vi "Run.vi"(8 "error in (no error)":errorcluster, 10 "반복":u32, 11 "Ch selection":T1) -> (0 "error out":errorcluster, 3 "stop":bool)   [LabVIEW 2019]
uses:
  _ctrl/rw.ctl
  cmd_runStop.ctl
  cmd_timer.ctl
  Durability/common/result.ctl
  _ctrl/init-r-stop.ctl
  Durability/common/Global 1.vi
  Glob_setting.vi
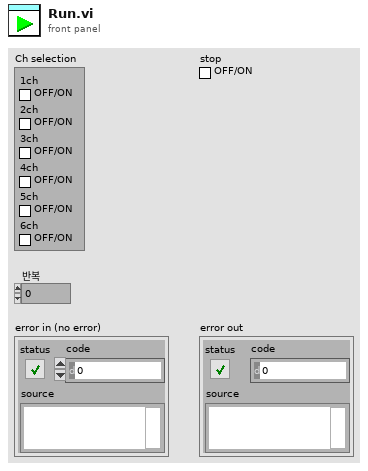
[diagram p1: front panel]
types:
  T1 = cluster{"1ch":bool, "2ch":bool, "3ch":bool, "4ch":bool, "5ch":bool, "6ch":bool}
  T2 = typedef "cmd_runStop.ctl" = enum16{"Init", "Run 1", "Stop", "Run 2", "Exit"}
  T3 = typedef "rw.ctl" = enum16{"read", "write"}
  T4 = typedef "cap_config.ctl" = cluster{"Test Mode":enum32{"6.3.2 저온 작동/방치 시험", "6.3.3 고온 작동/방치 시험", "6.3.4 온도 싸이클 시험", "6.3.6 온습도 싸이클 시험", "6.3.8 결로 시험", "6.3.9 빙결 시험"}, "ON time[ms]":dbl, "OFF time[ms]":dbl, "1. 작동시간[분]":dbl, "2. 미작동시간[분]":dbl, "3. 작동시간[분]":dbl, "level[V]":dbl, "duty":dbl, "Freq":dbl, "Voltage+[V]":dbl, "Voltage-[V]":dbl, "Current+[A]":dbl, "Current-[A]":dbl, "출력전압[V]":dbl, "출력전류[A]":dbl, "OVP Level":dbl, "OCP Level":dbl, "Time Div":u16, "Record Len":i32, "방전 기준[V]":dbl, "Repeate (Each Ch)":u32, "Cycle[N]":u32, "ON/OFF 회 수[N]":dbl, "TrigPos[%]":dbl, "시험시간[분]":dbl}
  T5 = enum32{"6.3.2 저온 작동/방치 시험", "6.3.3 고온 작동/방치 시험", "6.3.4 온도 싸이클 시험", "6.3.6 온습도 싸이클 시험", "6.3.8 결로 시험", "6.3.9 빙결 시험"}
  T6 = typedef "result.ctl" = enum16{"Init", "OK", "NG", "Shutdown", "Testing", "Completion", "Device Error", "Start", "작동", "미작동", "작동 대기", "작동 1"}
  T7 = typedef "cmd_timer.ctl" = enum16{"init", "init_update", "run", "default", "update"}
  T8 = typedef "init-r-stop.ctl" = enum16{"ini", "read", "stop"}
  T9 = typedef "rc-seq_enum.ctl" = enum16{"hw set", "Pwr-in on", "ch-relay on", "Pwr-out on", "AO on", "AO 0v", "Pwr-in off", "Relay-all off", "Pwr-out off", "Discharge", "950 read", "Run", "Stop"}
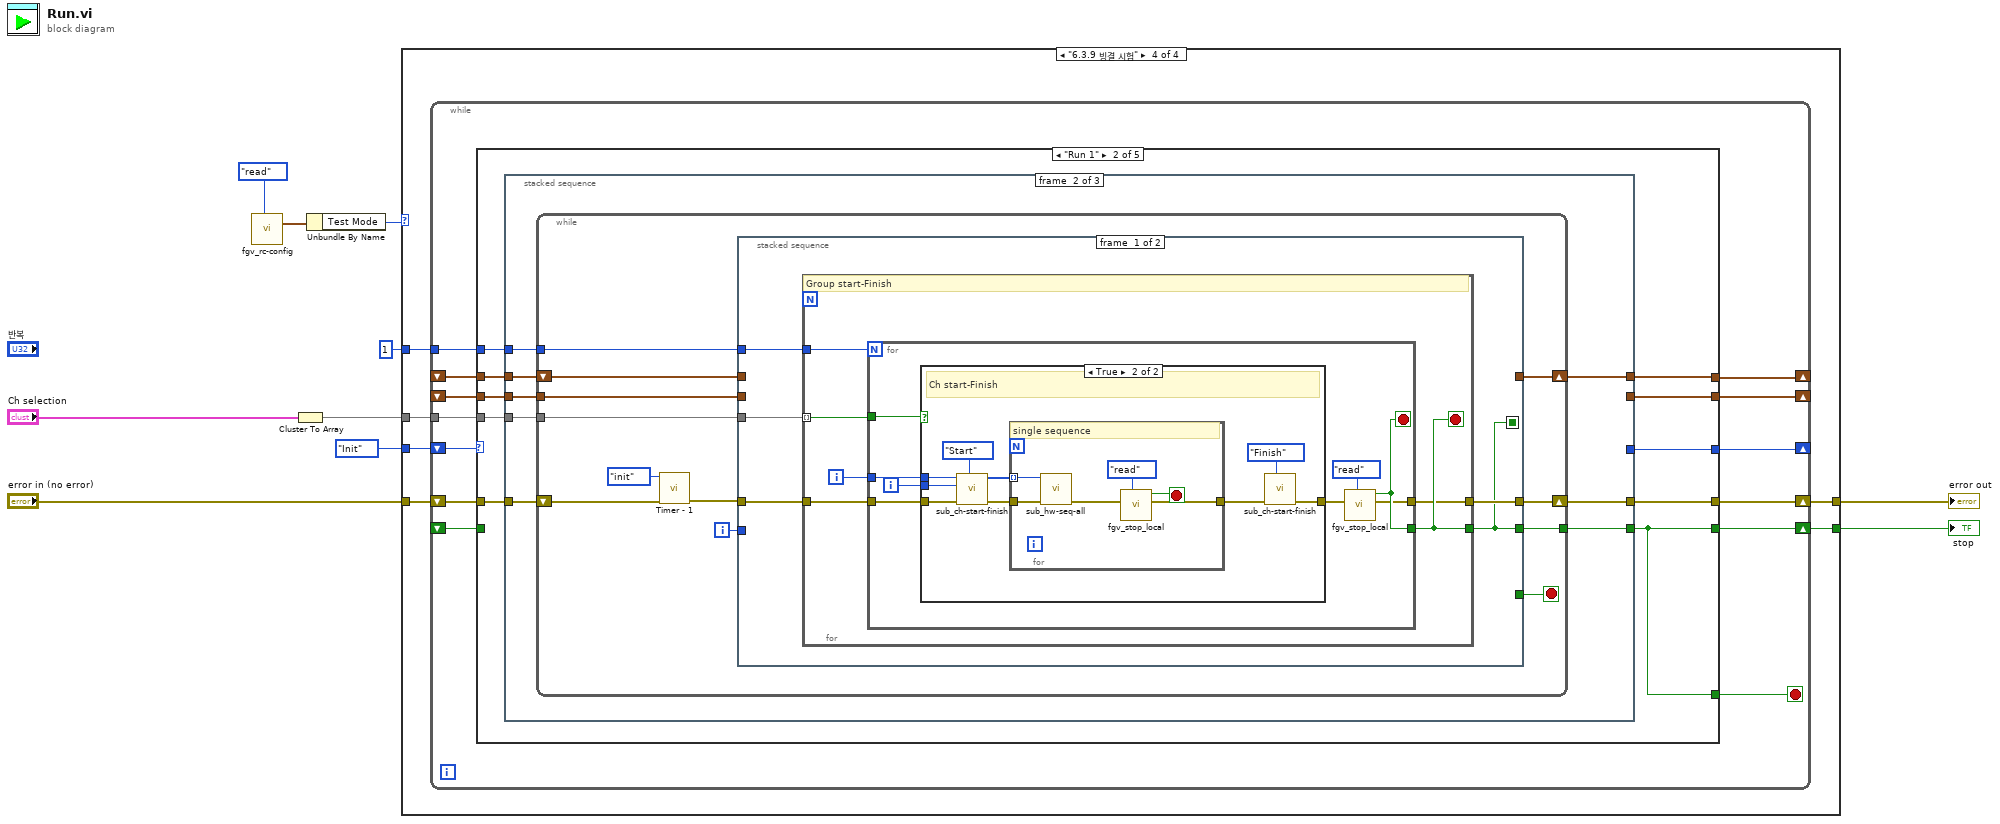
[diagram p0: block diagram]
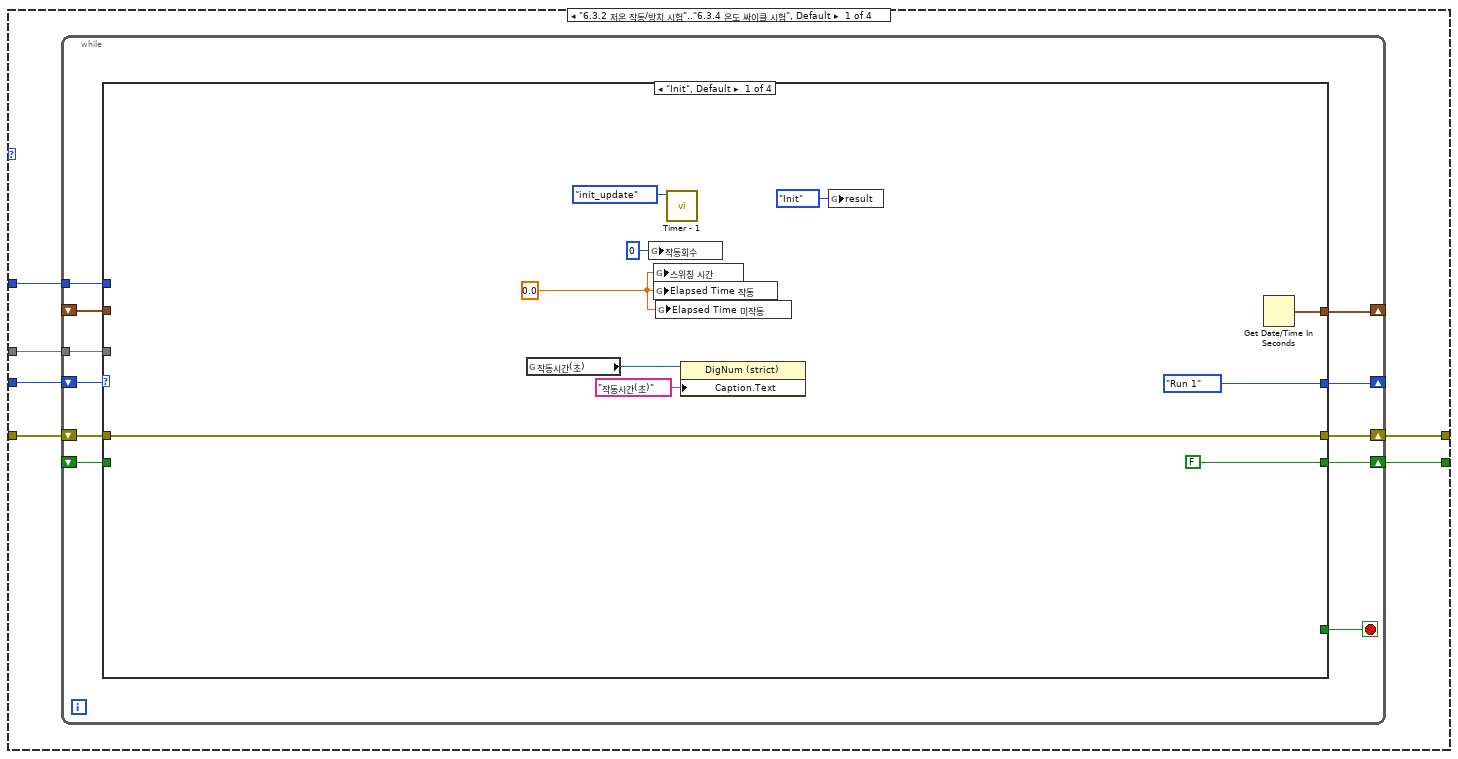
[diagram p2: hidden frame]
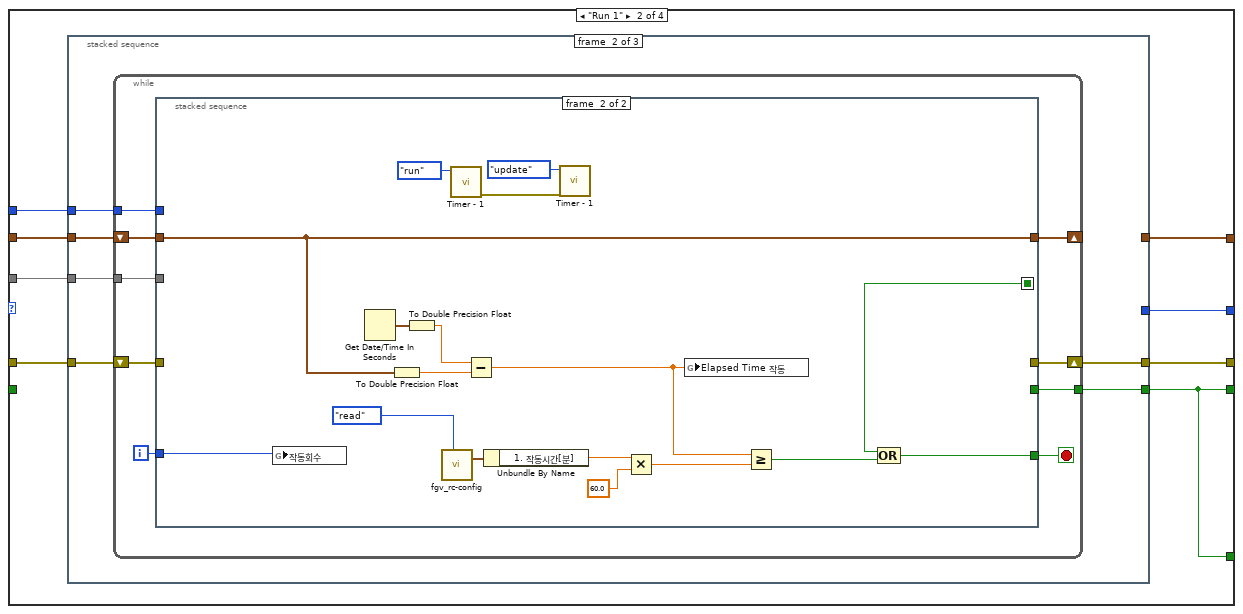
[diagram p3: hidden frame]
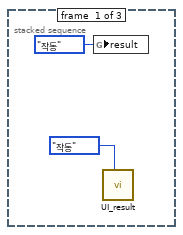
[diagram p4: hidden frame]
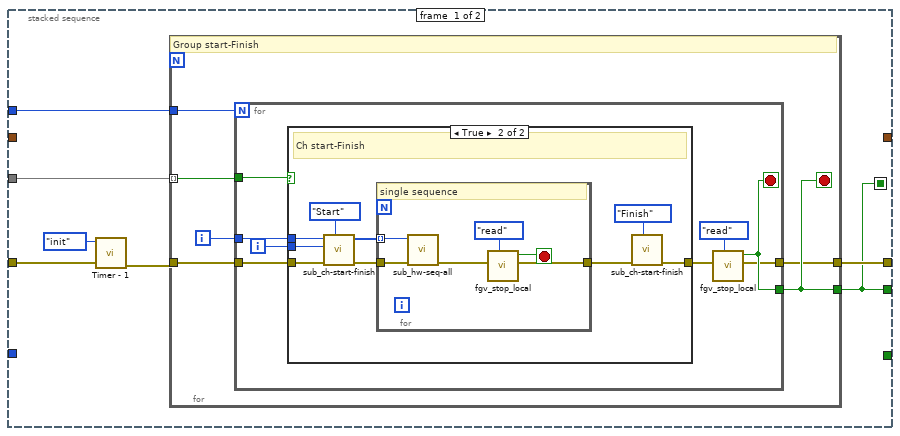
[diagram p5: hidden frame]
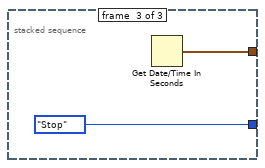
[diagram p7: hidden frame]
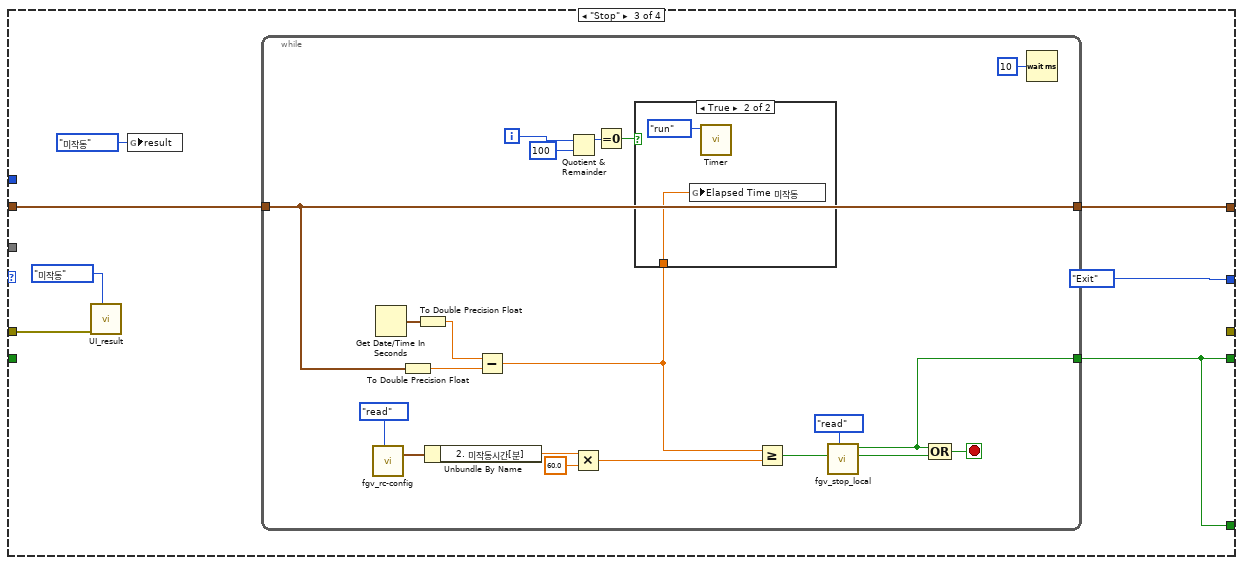
[diagram p8: hidden frame]
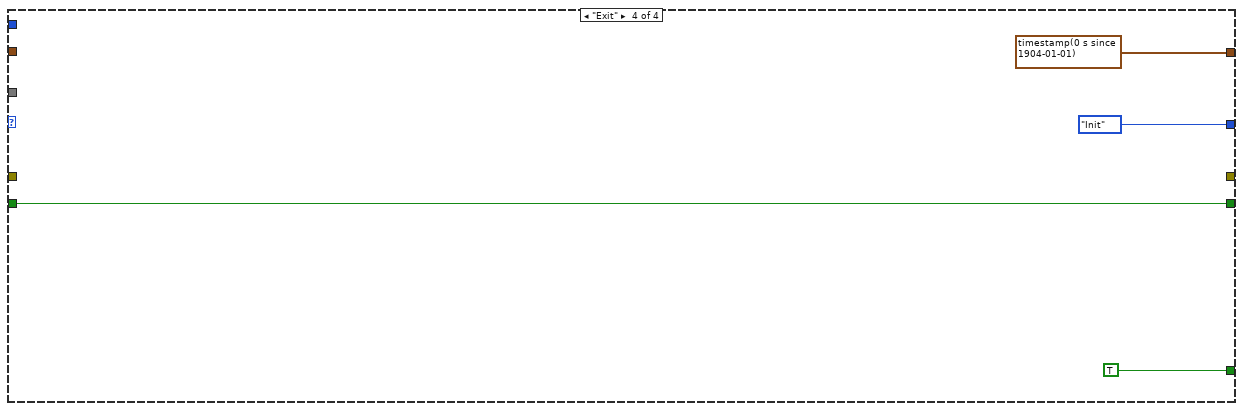
[diagram p10: hidden frame]
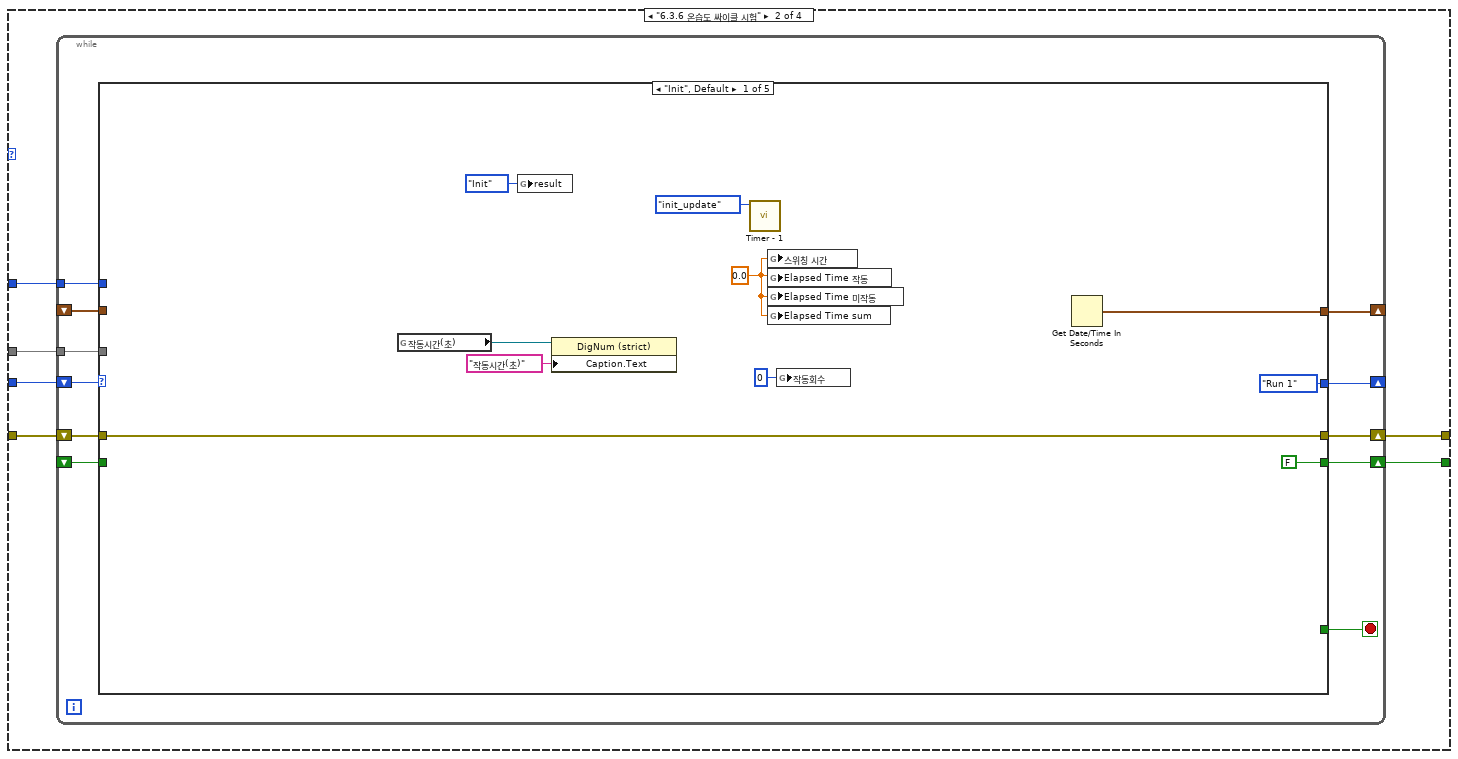
[diagram p11: hidden frame]
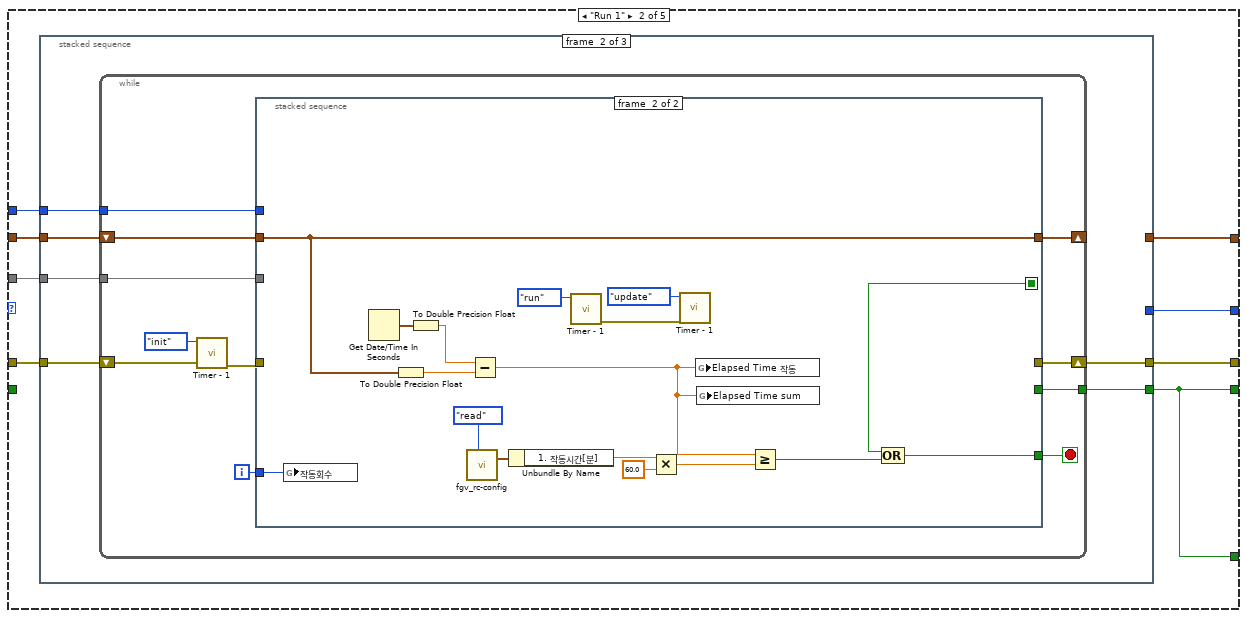
[diagram p12: hidden frame]
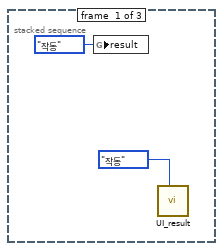
[diagram p13: hidden frame]
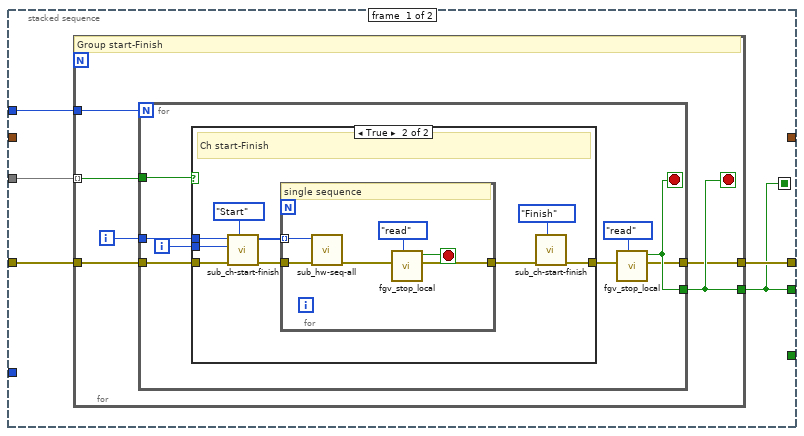
[diagram p14: hidden frame]
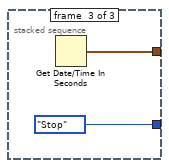
[diagram p16: hidden frame]
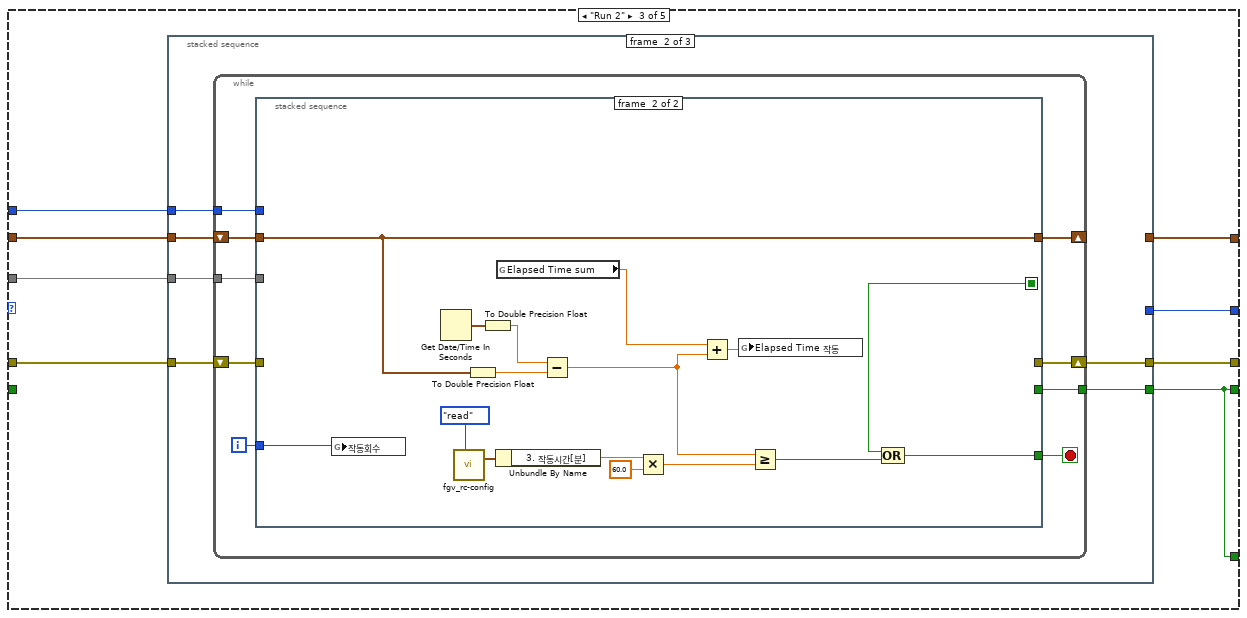
[diagram p17: hidden frame]
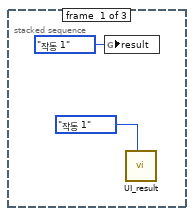
[diagram p18: hidden frame]
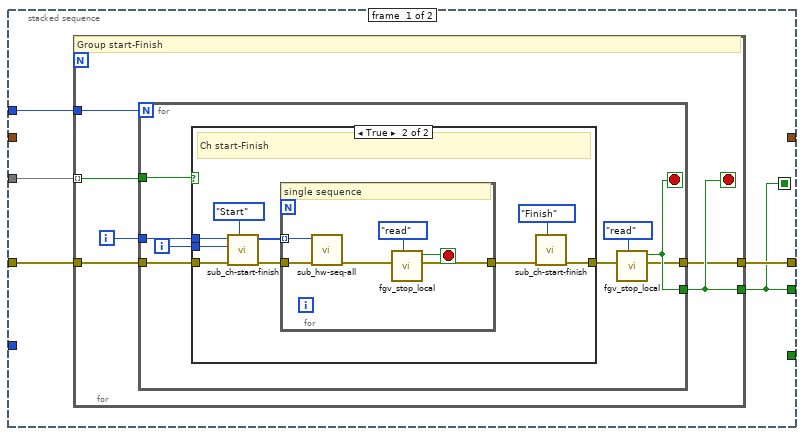
[diagram p19: hidden frame]
diagram:
  n1 = call "fgv_rc-config.vi"("cmd"=rw."read") -> ("Testconfig out"=w5:T4)  [unwired: 9 in, 1 out]
  n2 = Cluster To Array(cluster="Ch selection") -> (array=w6:bool[])
  n3 = Unbundle By Name(w5) -> ("Test Mode"=w3:T5)
  n4 = case shown="\"6.3.9 빙결 시험\"" w3 {
    tunnel: u32 1 ("반복") -> [w16 w156 w379 w637]
    tunnel: [w15 w155 w378 w636] -> w10
    tunnel: "error in (no error)" -> [w14 w154 w377 w635]
    tunnel: [w13 w153 w376 w634] -> w8
    tunnel: w6 -> [w12 w152 w375 w633]
    tunnel: cmd_runStop."Init" ("Enum") -> [w11 w151 w374 w632]
    frame "6.3.2 저온 작동/방치 시험".."6.3.4 온도 싸이클 시험", Default {
      n5 = while {
        tunnel: w16 -> [w27]
        tunnel: w12 -> [w23]
        shift-right: [w26] -> w15
        shift-left: w14 -> [w25]
        shift-right: [w21] -> _
        shift-left: _ -> [w20]
        shift-right: [w19] -> _
        shift-left: w11 -> [w22]
        shift-right: [w24] -> w13
        shift-left: _ -> [w18]
        stop <- w17 stop-if-true
        n6 = case shown="\"Init\", Default" w22 {
          tunnel: w27 -> [_ w45 _ _]
          tunnel: [w36 w44 _ _] -> w26
          tunnel: w25 -> [w36 w43 w121 _]
          tunnel: [FALSE ("stop") w38 w120 w148] -> w24
          tunnel: w23 -> [_ w42 _ _]
          tunnel: [w37 w40 w124 timestamp(0 s since 1904-01-01) ("seconds since 1Jan1904")] -> w21
          tunnel: w20 -> [_ w41 w125 _]
          tunnel: [cmd_runStop."Run 1" ("Enum") w39 cmd_runStop."Exit" ("Enum") cmd_runStop."Init" ("Enum")] -> w19
          tunnel: w18 -> [_ _ _ w148]
          tunnel: [_ w38 w120 TRUE] -> w17
          frame "Init", Default {
            w33 = 0.0 ("Elapsed Time")
            n7 = global read "Global 1.vi" "작동시간(초)"() -> (w31:refnum<vi>)
            n8 = global write "Global 1.vi" "작동회수"(0 ("작동회수")) -> ()
            n9 = global write "Global 1.vi" "스위칭 시간"(w33) -> ()
            n10 = global write "Global 1.vi" "Elapsed Time 작동"(w33) -> ()
            n11 = global write "Global 1.vi" "Elapsed Time 미작동"(w33) -> ()
            n12 = call "Timer - 1.vi"("cmd"=cmd_timer."init_update") -> ()  [unwired: 8 in, 3 out]
            n13 = property class="DigNum (strict)"(reference=w31, "Caption.Text"="작동시간(초)" ("Label.Text")) -> ()  [unwired: 1 in, 2 out]
            n14 = global write "Glob_setting.vi" "result"(result."Init" ("result")) -> ()
            n15 = Get Date/Time In Seconds() -> (seconds since 1Jan1904=w37:timestamp)
          }
          frame "Run 1" {
            n16 = stacked-sequence {
              tunnel: w45 -> [_ w53 _]
              tunnel: [_ w52 _] -> w44
              tunnel: w43 -> [_ w51 _]
              tunnel: [_ w50 _] -> w38
              tunnel: w42 -> [_ w49 _]
              tunnel: w41 -> [_ w48 _]
              tunnel: [_ _ w117] -> w40
              tunnel: [_ _ cmd_runStop."Stop" ("Enum")] -> w39
              frame #0 {
                n17 = global write "Glob_setting.vi" "result"(result."작동" ("result")) -> ()
                n18 = call "UI_result.vi"("result"=result."작동") -> ()  [unwired: 10 in, 1 out]
              }
              frame #1 {
                n19 = while {
                  tunnel: w53 -> [w62]
                  tunnel: [w59] -> w50
                  tunnel: w49 -> [w58]
                  shift-right: [w61] -> w52
                  shift-left: w51 -> [w60]
                  shift-right: [w55] -> _
                  shift-left: w48 -> [w57]
                  i -> [w54]
                  stop <- w56 stop-if-true
                  n20 = stacked-sequence {
                    seq-local: [w66 _] -> [_ w111]
                    tunnel: w62 -> [w69 _]
                    tunnel: [w68 _] -> w61
                    tunnel: w60 -> [w64 _]
                    tunnel: [w66 _] -> w59
                    tunnel: w58 -> [w67 _]
                    tunnel: w57 -> [_ w108]
                    tunnel: [_ w109] -> w56
                    tunnel: [_ w108] -> w55
                    tunnel: w54 -> [_ w104]
                    frame #0 {
                      n21 = call "Timer - 1.vi"("error in (no error)"=w64, "cmd"=cmd_timer."init") -> ("error out"=w63:errorcluster)  [unwired: 7 in, 2 out]
                      n22 = for {
                        tunnel: [w73] -> w66
                        tunnel: w67 -> [w75] mode=indexing
                        tunnel: w63 -> [w71]
                        tunnel: [w72] -> w68
                        tunnel: w69 -> [w70]
                        i -> [w74]
                        stop <- w73 stop-if-true
                        # "Group start-Finish"
                        n23 = for {
                          N: w70 -> [_]
                          tunnel: w74 -> [w82]
                          tunnel: w71 -> [w81]
                          tunnel: [w76] -> w72
                          tunnel: w75 -> [w83]
                          tunnel: [w77] -> w73
                          i -> [w80]
                          stop <- w77 stop-if-true
                          n24 = case shown="True" w83 {
                            tunnel: w82 -> [_ w92]
                            tunnel: [w84 w85] -> w78
                            tunnel: w81 -> [w84 w87]
                            tunnel: w80 -> [_ w86]
                            frame False {
                            }
                            frame True {
                              # "Ch start-Finish"
                              n25 = call "sub_ch-start-finish.vi"("cmd"=enum16{"Start", "Finish"}."Start", "error in"=w87, "repeat"=w86, "Ch"=w92) -> ("error out"=w93:errorcluster, "HWseq-array"=w90:T9[])  [unwired: 5 in, 1 out]
                              n26 = for {
                                tunnel: w90 -> [w97] mode=indexing
                                tunnel: w93 -> [w94]
                                tunnel: [w95] -> w88
                                stop <- w98 stop-if-true
                                # "single sequence"
                                n27 = call "sub_hw-seq-all.vi"("error"=w94, "HWseq"=w97) -> ("error out"=w96:errorcluster)  [unwired: 9 in]
                                n28 = call "fgv_stop_local.vi"("cmd"=init-r-stop."read", "error in (no error)"=w96) -> ("error out"=w95:errorcluster, "stop"=w98:bool)  [unwired: 8 in]
                              }
                              n29 = call "sub_ch-start-finish.vi"("cmd"=enum16{"Start", "Finish"}."Finish", "error in"=w88) -> ("error out"=w85:errorcluster)  [unwired: 7 in, 2 out]
                            }
                          }
                          n30 = call "fgv_stop_local.vi"("cmd"=init-r-stop."read", "error in (no error)"=w78) -> ("error out"=w76:errorcluster, "stop"=w77:bool)  [unwired: 8 in]
                        }
                      }
                    }
                    frame #1 {
                      n31 = global write "Global 1.vi" "작동회수"(w104) -> ()
                      n32 = Get Date/Time In Seconds() -> (seconds since 1Jan1904=w116:timestamp)
                      n33 = To Double Precision Float(number=w108) -> (double precision float=w114:dbl)
                      n34 = To Double Precision Float(number=w116) -> (double precision float=w115:dbl)
                      n35 = call "fgv_rc-config.vi"("cmd"=rw."read") -> ("Testconfig out"=w113:T4)  [unwired: 9 in, 1 out]
                      n36 = call "Timer - 1.vi"("cmd"=cmd_timer."run") -> ("error out"=w100:errorcluster)  [unwired: 8 in, 2 out]
                      n37 = Subtract(x=w115, y=w114) -> (x-y=w103:dbl)
                      n38 = Unbundle By Name(w113) -> ("1. 작동시간[분]"=w107:dbl)
                      n39 = call "Timer - 1.vi"("error in (no error)"=w100, "cmd"=cmd_timer."update") -> ()  [unwired: 7 in, 3 out]
                      n40 = Multiply(x=w107, y=60.0) -> (x*y=w105:dbl)
                      n41 = global write "Global 1.vi" "Elapsed Time 작동"(w103) -> ()
                      n42 = Greater Or Equal?(x=w103, y=w105) -> (x >= y?=w110:bool)
                      n43 = Compound Arithmetic op=OR(w111, w110) -> (w109:bool)
                    }
                  }
                }
              }
              frame #2 {
                n44 = Get Date/Time In Seconds() -> (seconds since 1Jan1904=w117:timestamp)
              }
            }
          }
          frame "Stop" {
            n45 = call "UI_result.vi"("result"=result."미작동", "error in (no error)"=w121) -> ()  [unwired: 9 in, 1 out]
            n46 = global write "Glob_setting.vi" "result"(result."미작동" ("result")) -> ()
            n47 = while {
              tunnel: w125 -> [w132]
              tunnel: [w132] -> w124
              tunnel: [w131] -> w120
              i -> [w127]
              stop <- w133 stop-if-true
              n48 = call "fgv_rc-config.vi"("cmd"=rw."read") -> ("Testconfig out"=w139:T4)  [unwired: 9 in, 1 out]
              n49 = Get Date/Time In Seconds() -> (seconds since 1Jan1904=w142:timestamp)
              n50 = To Double Precision Float(number=w132) -> (double precision float=w140:dbl)
              n51 = To Double Precision Float(number=w142) -> (double precision float=w141:dbl)
              n52 = Unbundle By Name(w139) -> ("2. 미작동시간[분]"=w137:dbl)
              n53 = Subtract(x=w141, y=w140) -> (x-y=w126:dbl)
              n54 = Quotient & Remainder(x=w127, y=100) -> (x-y*floor(x/y)=w129:i32)  [unwired: 1 out]
              n55 = Multiply(x=w137, y=60.0) -> (x*y=w135:dbl)
              n56 = Equal To 0?(x=w129) -> (x = 0?=w128:bool)
              n57 = case shown="True" w128 {
                tunnel: w126 -> [_ w145]
                frame False {
                }
                frame True {
                  n58 = global write "Global 1.vi" "Elapsed Time 미작동"(w145) -> ()
                  n59 = call "Timer.vi"("cmd"=cmd_timer."run") -> ()  [unwired: 8 in, 3 out]
                }
              }
              n60 = Greater Or Equal?(x=w126, y=w135) -> (x >= y?=w134:bool)
              n61 = call "fgv_stop_local.vi"("cmd"=init-r-stop."read") -> ("stop"=w131:bool)  [unwired: 9 in, 1 out]
              n62 = Compound Arithmetic op=OR(w131, w134) -> (w133:bool)
              n63 = Wait (ms)(milliseconds to wait=u32 10) -> ()  [unwired: 1 out]
            }
          }
          frame "Exit" {
          }
        }
      }
    }
    frame "6.3.6 온습도 싸이클 시험" {
      n64 = while {
        tunnel: w156 -> [w167]
        tunnel: w152 -> [w163]
        shift-right: [w166] -> w155
        shift-left: w154 -> [w165]
        shift-right: [w161] -> _
        shift-left: _ -> [w160]
        shift-right: [w159] -> _
        shift-left: w151 -> [w162]
        shift-right: [w164] -> w153
        shift-left: _ -> [w158]
        stop <- w157 stop-if-true
        n65 = case shown="\"Init\", Default" w162 {
          tunnel: w167 -> [_ w185 w266 _ _]
          tunnel: [w176 w184 w265 _ _] -> w166
          tunnel: w165 -> [w176 w183 w264 w339 _]
          tunnel: [FALSE ("stop") w178 w259 w338 w371] -> w164
          tunnel: w163 -> [_ w182 w263 _ _]
          tunnel: [w177 w180 w261 w342 timestamp(0 s since 1904-01-01) ("seconds since 1Jan1904")] -> w161
          tunnel: w160 -> [_ w181 w262 w343 _]
          tunnel: [cmd_runStop."Run 1" ("Enum") w179 w260 w341 cmd_runStop."Init" ("Enum")] -> w159
          tunnel: w158 -> [_ _ _ _ w371]
          tunnel: [_ w178 w259 w338 TRUE] -> w157
          frame "Init", Default {
            w168 = 0.0 ("Elapsed Time")
            n66 = global read "Global 1.vi" "작동시간(초)"() -> (w172:refnum<vi>)
            n67 = global write "Glob_setting.vi" "result"(result."Init" ("result")) -> ()
            n68 = property class="DigNum (strict)"(reference=w172, "Caption.Text"="작동시간(초)" ("Label.Text")) -> ()  [unwired: 1 in, 2 out]
            n69 = call "Timer - 1.vi"("cmd"=cmd_timer."init_update") -> ()  [unwired: 8 in, 3 out]
            n70 = global write "Global 1.vi" "스위칭 시간"(w168) -> ()
            n71 = global write "Global 1.vi" "Elapsed Time 작동"(w168) -> ()
            n72 = global write "Global 1.vi" "Elapsed Time 미작동"(w168) -> ()
            n73 = global write "Global 1.vi" "Elapsed Time sum"(w168) -> ()
            n74 = global write "Global 1.vi" "작동회수"(0 ("작동회수")) -> ()
            n75 = Get Date/Time In Seconds() -> (seconds since 1Jan1904=w177:timestamp)
          }
          frame "Run 1" {
            n76 = stacked-sequence {
              tunnel: w185 -> [_ w193 _]
              tunnel: [_ w192 _] -> w184
              tunnel: w183 -> [_ w191 _]
              tunnel: [_ w190 _] -> w178
              tunnel: w182 -> [_ w189 _]
              tunnel: w181 -> [_ w188 _]
              tunnel: [_ _ w257] -> w180
              tunnel: [_ _ cmd_runStop."Stop" ("Enum")] -> w179
              frame #0 {
                n77 = global write "Glob_setting.vi" "result"(result."작동" ("result")) -> ()
                n78 = call "UI_result.vi"("result"=result."작동") -> ()  [unwired: 10 in, 1 out]
              }
              frame #1 {
                n79 = while {
                  tunnel: w193 -> [w204]
                  tunnel: [w202] -> w190
                  tunnel: w189 -> [w201]
                  shift-right: [w203] -> w192
                  shift-left: w191 -> [w195]
                  shift-right: [w198] -> _
                  shift-left: w188 -> [w200]
                  i -> [w197]
                  stop <- w199 stop-if-true
                  n80 = call "Timer - 1.vi"("error in (no error)"=w195, "cmd"=cmd_timer."init") -> ("error out"=w194:errorcluster)  [unwired: 7 in, 2 out]
                  n81 = stacked-sequence {
                    seq-local: [w205 _] -> [_ w251]
                    tunnel: w204 -> [w209 _]
                    tunnel: [w208 _] -> w203
                    tunnel: w194 -> [w207 _]
                    tunnel: [w205 _] -> w202
                    tunnel: w201 -> [w206 _]
                    tunnel: w200 -> [_ w248]
                    tunnel: [_ w249] -> w199
                    tunnel: [_ w248] -> w198
                    tunnel: w197 -> [_ w244]
                    frame #0 {
                      n82 = for {
                        tunnel: [w213] -> w205
                        tunnel: w206 -> [w215] mode=indexing
                        tunnel: w207 -> [w211]
                        tunnel: [w212] -> w208
                        tunnel: w209 -> [w210]
                        i -> [w214]
                        stop <- w213 stop-if-true
                        # "Group start-Finish"
                        n83 = for {
                          N: w210 -> [_]
                          tunnel: w214 -> [w222]
                          tunnel: w211 -> [w221]
                          tunnel: [w216] -> w212
                          tunnel: w215 -> [w223]
                          tunnel: [w217] -> w213
                          i -> [w220]
                          stop <- w217 stop-if-true
                          n84 = case shown="True" w223 {
                            tunnel: w222 -> [_ w232]
                            tunnel: [w224 w225] -> w218
                            tunnel: w221 -> [w224 w227]
                            tunnel: w220 -> [_ w226]
                            frame False {
                            }
                            frame True {
                              # "Ch start-Finish"
                              n85 = call "sub_ch-start-finish.vi"("cmd"=enum16{"Start", "Finish"}."Start", "error in"=w227, "repeat"=w226, "Ch"=w232) -> ("error out"=w233:errorcluster, "HWseq-array"=w230:T9[])  [unwired: 5 in, 1 out]
                              n86 = for {
                                tunnel: w230 -> [w237] mode=indexing
                                tunnel: w233 -> [w234]
                                tunnel: [w235] -> w228
                                stop <- w238 stop-if-true
                                # "single sequence"
                                n87 = call "sub_hw-seq-all.vi"("error"=w234, "HWseq"=w237) -> ("error out"=w236:errorcluster)  [unwired: 9 in]
                                n88 = call "fgv_stop_local.vi"("cmd"=init-r-stop."read", "error in (no error)"=w236) -> ("error out"=w235:errorcluster, "stop"=w238:bool)  [unwired: 8 in]
                              }
                              n89 = call "sub_ch-start-finish.vi"("cmd"=enum16{"Start", "Finish"}."Finish", "error in"=w228) -> ("error out"=w225:errorcluster)  [unwired: 7 in, 2 out]
                            }
                          }
                          n90 = call "fgv_stop_local.vi"("cmd"=init-r-stop."read", "error in (no error)"=w218) -> ("error out"=w216:errorcluster, "stop"=w217:bool)  [unwired: 8 in]
                        }
                      }
                    }
                    frame #1 {
                      n91 = global write "Global 1.vi" "작동회수"(w244) -> ()
                      n92 = Get Date/Time In Seconds() -> (seconds since 1Jan1904=w256:timestamp)
                      n93 = To Double Precision Float(number=w248) -> (double precision float=w254:dbl)
                      n94 = To Double Precision Float(number=w256) -> (double precision float=w255:dbl)
                      n95 = call "fgv_rc-config.vi"("cmd"=rw."read") -> ("Testconfig out"=w253:T4)  [unwired: 9 in, 1 out]
                      n96 = Subtract(x=w255, y=w254) -> (x-y=w240:dbl)
                      n97 = Unbundle By Name(w253) -> ("1. 작동시간[분]"=w247:dbl)
                      n98 = call "Timer - 1.vi"("cmd"=cmd_timer."run") -> ("error out"=w241:errorcluster)  [unwired: 8 in, 2 out]
                      n99 = Multiply(x=w247, y=60.0) -> (x*y=w245:dbl)
                      n100 = call "Timer - 1.vi"("error in (no error)"=w241, "cmd"=cmd_timer."update") -> ()  [unwired: 7 in, 3 out]
                      n101 = global write "Global 1.vi" "Elapsed Time 작동"(w240) -> ()
                      n102 = global write "Global 1.vi" "Elapsed Time sum"(w240) -> ()
                      n103 = Greater Or Equal?(x=w240, y=w245) -> (x >= y?=w250:bool)
                      n104 = Compound Arithmetic op=OR(w251, w250) -> (w249:bool)
                    }
                  }
                }
              }
              frame #2 {
                n105 = Get Date/Time In Seconds() -> (seconds since 1Jan1904=w257:timestamp)
              }
            }
          }
          frame "Run 2" {
            n106 = stacked-sequence {
              tunnel: w266 -> [_ w274 _]
              tunnel: [_ w273 _] -> w265
              tunnel: w264 -> [_ w272 _]
              tunnel: [_ w271 _] -> w259
              tunnel: w263 -> [_ w270 _]
              tunnel: w262 -> [_ w269 _]
              tunnel: [_ _ w335] -> w261
              tunnel: [_ _ cmd_runStop."Exit" ("Enum")] -> w260
              frame #0 {
                n107 = global write "Glob_setting.vi" "result"(result."작동 1" ("result")) -> ()
                n108 = call "UI_result.vi"("result"=result."작동 1") -> ()  [unwired: 10 in, 1 out]
              }
              frame #1 {
                n109 = while {
                  tunnel: w274 -> [w283]
                  tunnel: [w280] -> w271
                  tunnel: w270 -> [w279]
                  shift-right: [w282] -> w273
                  shift-left: w272 -> [w281]
                  shift-right: [w276] -> _
                  shift-left: w269 -> [w278]
                  i -> [w275]
                  stop <- w277 stop-if-true
                  n110 = stacked-sequence {
                    seq-local: [w284 _] -> [_ w329]
                    tunnel: w283 -> [w288 _]
                    tunnel: [w287 _] -> w282
                    tunnel: w281 -> [w286 _]
                    tunnel: [w284 _] -> w280
                    tunnel: w279 -> [w285 _]
                    tunnel: w278 -> [_ w326]
                    tunnel: [_ w327] -> w277
                    tunnel: [_ w326] -> w276
                    tunnel: w275 -> [_ w322]
                    frame #0 {
                      n111 = for {
                        tunnel: [w292] -> w284
                        tunnel: w285 -> [w294] mode=indexing
                        tunnel: w286 -> [w290]
                        tunnel: [w291] -> w287
                        tunnel: w288 -> [w289]
                        i -> [w293]
                        stop <- w292 stop-if-true
                        # "Group start-Finish"
                        n112 = for {
                          N: w289 -> [_]
                          tunnel: w293 -> [w301]
                          tunnel: w290 -> [w300]
                          tunnel: [w295] -> w291
                          tunnel: w294 -> [w302]
                          tunnel: [w296] -> w292
                          i -> [w299]
                          stop <- w296 stop-if-true
                          n113 = case shown="True" w302 {
                            tunnel: w301 -> [_ w311]
                            tunnel: [w303 w304] -> w297
                            tunnel: w300 -> [w303 w306]
                            tunnel: w299 -> [_ w305]
                            frame False {
                            }
                            frame True {
                              # "Ch start-Finish"
                              n114 = call "sub_ch-start-finish.vi"("cmd"=enum16{"Start", "Finish"}."Start", "error in"=w306, "repeat"=w305, "Ch"=w311) -> ("error out"=w312:errorcluster, "HWseq-array"=w309:T9[])  [unwired: 5 in, 1 out]
                              n115 = for {
                                tunnel: w309 -> [w316] mode=indexing
                                tunnel: w312 -> [w313]
                                tunnel: [w314] -> w307
                                stop <- w317 stop-if-true
                                # "single sequence"
                                n116 = call "sub_hw-seq-all.vi"("error"=w313, "HWseq"=w316) -> ("error out"=w315:errorcluster)  [unwired: 9 in]
                                n117 = call "fgv_stop_local.vi"("cmd"=init-r-stop."read", "error in (no error)"=w315) -> ("error out"=w314:errorcluster, "stop"=w317:bool)  [unwired: 8 in]
                              }
                              n118 = call "sub_ch-start-finish.vi"("cmd"=enum16{"Start", "Finish"}."Finish", "error in"=w307) -> ("error out"=w304:errorcluster)  [unwired: 7 in, 2 out]
                            }
                          }
                          n119 = call "fgv_stop_local.vi"("cmd"=init-r-stop."read", "error in (no error)"=w297) -> ("error out"=w295:errorcluster, "stop"=w296:bool)  [unwired: 8 in]
                        }
                      }
                    }
                    frame #1 {
                      n120 = global write "Global 1.vi" "작동회수"(w322) -> ()
                      n121 = Get Date/Time In Seconds() -> (seconds since 1Jan1904=w334:timestamp)
                      n122 = call "fgv_rc-config.vi"("cmd"=rw."read") -> ("Testconfig out"=w331:T4)  [unwired: 9 in, 1 out]
                      n123 = To Double Precision Float(number=w326) -> (double precision float=w332:dbl)
                      n124 = To Double Precision Float(number=w334) -> (double precision float=w333:dbl)
                      n125 = Unbundle By Name(w331) -> ("3. 작동시간[분]"=w325:dbl)
                      n126 = global read "Global 1.vi" "Elapsed Time sum"() -> (w320:dbl)
                      n127 = Subtract(x=w333, y=w332) -> (x-y=w321:dbl)
                      n128 = Multiply(x=w325, y=60.0) -> (x*y=w323:dbl)
                      n129 = Add(x=w320, y=w321) -> (x+y=w319:dbl)
                      n130 = global write "Global 1.vi" "Elapsed Time 작동"(w319) -> ()
                      n131 = Greater Or Equal?(x=w321, y=w323) -> (x >= y?=w328:bool)
                      n132 = Compound Arithmetic op=OR(w329, w328) -> (w327:bool)
                    }
                  }
                }
              }
              frame #2 {
                n133 = Get Date/Time In Seconds() -> (seconds since 1Jan1904=w335:timestamp)
              }
            }
          }
          frame "Stop" {
            n134 = global write "Glob_setting.vi" "result"(result."미작동" ("result")) -> ()
            n135 = call "UI_result.vi"("result"=result."미작동", "error in (no error)"=w339) -> ()  [unwired: 9 in, 1 out]
            n136 = stacked-sequence {
              tunnel: w343 -> [w345 _]
              tunnel: [_ w368] -> w342
              tunnel: [w344 _] -> w338
              tunnel: [_ cmd_runStop."Run 2" ("Enum")] -> w341
              frame #0 {
                n137 = while {
                  tunnel: [w351] -> w344
                  shift-right: [w352] -> _
                  shift-left: w345 -> [w352]
                  i -> [w347]
                  stop <- w353 stop-if-true
                  n138 = call "fgv_rc-config.vi"("cmd"=rw."read") -> ("Testconfig out"=w359:T4)  [unwired: 9 in, 1 out]
                  n139 = Get Date/Time In Seconds() -> (seconds since 1Jan1904=w362:timestamp)
                  n140 = To Double Precision Float(number=w352) -> (double precision float=w360:dbl)
                  n141 = To Double Precision Float(number=w362) -> (double precision float=w361:dbl)
                  n142 = Unbundle By Name(w359) -> ("2. 미작동시간[분]"=w357:dbl)
                  n143 = Quotient & Remainder(x=w347, y=100) -> (x-y*floor(x/y)=w349:i32)  [unwired: 1 out]
                  n144 = Subtract(x=w361, y=w360) -> (x-y=w346:dbl)
                  n145 = Equal To 0?(x=w349) -> (x = 0?=w348:bool)
                  n146 = case shown="True" w348 {
                    tunnel: w346 -> [_ w365]
                    frame False {
                    }
                    frame True {
                      n147 = global write "Global 1.vi" "Elapsed Time 미작동"(w365) -> ()
                      n148 = call "Timer.vi"("cmd"=cmd_timer."run") -> ()  [unwired: 8 in, 3 out]
                    }
                  }
                  n149 = Multiply(x=w357, y=60.0) -> (x*y=w355:dbl)
                  n150 = Greater Or Equal?(x=w346, y=w355) -> (x >= y?=w354:bool)
                  n151 = call "fgv_stop_local.vi"("cmd"=init-r-stop."read") -> ("stop"=w351:bool)  [unwired: 9 in, 1 out]
                  n152 = Compound Arithmetic op=OR(w351, w354) -> (w353:bool)
                  n153 = Wait (ms)(milliseconds to wait=u32 10) -> ()  [unwired: 1 out]
                }
              }
              frame #1 {
                n154 = disable-structure shown="Disabled" {
                  frame Disabled {
                    n155 = global write "Global 1.vi" "Elapsed Time 작동"(0.0 ("Elapsed Time")) -> ()
                  }
                  frame Enabled {
                  }
                }
                n156 = Get Date/Time In Seconds() -> (seconds since 1Jan1904=w368:timestamp)
              }
            }
          }
          frame "Exit" {
          }
        }
      }
    }
    frame "6.3.8 결로 시험" {
      n157 = while {
        tunnel: w379 -> [w392]
        tunnel: w375 -> [w388]
        shift-right: [w391] -> w378
        shift-left: w377 -> [w390]
        shift-right: [w386] -> _
        shift-left: _ -> [w385]
        shift-right: [w384] -> _
        shift-left: w374 -> [w387]
        shift-right: [w389] -> w376
        shift-left: _ -> [w383]
        shift-right: [w381] -> _
        shift-left: _ -> [w380]
        stop <- w382 stop-if-true
        n158 = case shown="\"Stop\"" w387 {
          tunnel: w392 -> [_ w414 w501 _ _]
          tunnel: [w402 w413 w500 _ _] -> w391
          tunnel: w390 -> [w402 w404 w499 w577 _]
          tunnel: [FALSE ("stop") w406 w492 w576 w630] -> w389
          tunnel: w388 -> [_ w412 w498 _ _]
          tunnel: [w399 w410 w496 w582 w628] -> w386
          tunnel: w385 -> [_ w411 w497 w583 _]
          tunnel: [cmd_runStop."Run 1" ("Enum") w409 w495 w581 cmd_runStop."Init" ("Enum")] -> w384
          tunnel: w383 -> [_ _ _ _ w630]
          tunnel: [_ w406 w492 w576 TRUE] -> w382
          tunnel: [w399 w407 w494 w579 w628] -> w381
          tunnel: w380 -> [_ w408 w493 w580 _]
          frame "Init", Default {
            w393 = 0.0 ("Elapsed Time")
            n159 = global write "Glob_setting.vi" "result"(result."Init" ("result")) -> ()
            n160 = global read "Global 1.vi" "작동시간(초)"() -> (w397:refnum<vi>)
            n161 = global write "Global 1.vi" "작동회수"(0 ("작동회수")) -> ()
            n162 = global write "Global 1.vi" "스위칭 시간"(w393) -> ()
            n163 = global write "Global 1.vi" "Elapsed Time 작동"(w393) -> ()
            n164 = global write "Global 1.vi" "Elapsed Time 미작동"(w393) -> ()
            n165 = global write "Global 1.vi" "ETime 작동대기"(w393) -> ()
            n166 = property class="DigNum (strict)"(reference=w397, "Caption.Text"="작동경과 시간(초)" ("Label.Text")) -> ()  [unwired: 1 in, 2 out]
            n167 = call "Timer - 1.vi"("cmd"=cmd_timer."init_update") -> ()  [unwired: 8 in, 3 out]
            n168 = Get Date/Time In Seconds() -> (seconds since 1Jan1904=w399:timestamp)
          }
          frame "Run 1" {
            n169 = call "Timer - 1.vi"("error in (no error)"=w404, "cmd"=cmd_timer."init") -> ("error out"=w403:errorcluster)  [unwired: 7 in, 2 out]
            n170 = stacked-sequence {
              tunnel: w414 -> [_ w424 _]
              tunnel: [_ w423 _] -> w413
              tunnel: w403 -> [_ w422 _]
              tunnel: [_ w421 _] -> w406
              tunnel: w412 -> [_ w420 _]
              tunnel: w411 -> [_ w419 _]
              tunnel: [_ w418 _] -> w410
              tunnel: [_ _ cmd_runStop."Stop" ("Enum")] -> w409
              tunnel: w408 -> [_ w417 w490]
              tunnel: [_ _ w490] -> w407
              frame #0 {
                n171 = global write "Glob_setting.vi" "result"(result."작동" ("result")) -> ()
                n172 = call "UI_result.vi"("result"=result."작동") -> ()  [unwired: 10 in, 1 out]
              }
              frame #1 {
                n173 = while {
                  tunnel: w424 -> [w434]
                  tunnel: [w431] -> w421
                  tunnel: w420 -> [w430]
                  shift-right: [w433] -> w423
                  shift-left: w422 -> [w432]
                  shift-right: [w427] -> w418
                  shift-left: w419 -> [w429]
                  tunnel: w417 -> [w425]
                  i -> [w426]
                  stop <- w428 stop-if-true
                  n174 = stacked-sequence {
                    seq-local: [w435 _] -> [_ w481]
                    tunnel: w434 -> [w439 _]
                    tunnel: [w438 _] -> w433
                    tunnel: w432 -> [w437 _]
                    tunnel: [w435 _] -> w431
                    tunnel: w430 -> [w436 _]
                    tunnel: w429 -> [_ w478]
                    tunnel: [_ w487] -> w428
                    tunnel: [_ w478] -> w427
                    tunnel: w426 -> [_ w482]
                    tunnel: w425 -> [_ w473]
                    frame #0 {
                      n175 = for {
                        tunnel: [w443] -> w435
                        tunnel: w436 -> [w445] mode=indexing
                        tunnel: w437 -> [w441]
                        tunnel: [w442] -> w438
                        tunnel: w439 -> [w440]
                        i -> [w444]
                        stop <- w443 stop-if-true
                        # "Group start-Finish"
                        n176 = for {
                          N: w440 -> [_]
                          tunnel: w444 -> [w452]
                          tunnel: w441 -> [w451]
                          tunnel: [w446] -> w442
                          tunnel: w445 -> [w453]
                          tunnel: [w447] -> w443
                          i -> [w450]
                          stop <- w447 stop-if-true
                          n177 = case shown="True" w453 {
                            tunnel: w452 -> [_ w462]
                            tunnel: [w454 w455] -> w448
                            tunnel: w451 -> [w454 w457]
                            tunnel: w450 -> [_ w456]
                            frame False {
                            }
                            frame True {
                              # "Ch start-Finish"
                              n178 = call "sub_ch-start-finish.vi"("cmd"=enum16{"Start", "Finish"}."Start", "error in"=w457, "repeat"=w456, "Ch"=w462) -> ("error out"=w463:errorcluster, "HWseq-array"=w460:T9[])  [unwired: 5 in, 1 out]
                              n179 = for {
                                tunnel: w460 -> [w467] mode=indexing
                                tunnel: w463 -> [w464]
                                tunnel: [w465] -> w458
                                stop <- w468 stop-if-true
                                # "single sequence"
                                n180 = call "sub_hw-seq-all.vi"("error"=w464, "HWseq"=w467) -> ("error out"=w466:errorcluster)  [unwired: 9 in]
                                n181 = call "fgv_stop_local.vi"("cmd"=init-r-stop."read", "error in (no error)"=w466) -> ("error out"=w465:errorcluster, "stop"=w468:bool)  [unwired: 8 in]
                              }
                              n182 = call "sub_ch-start-finish.vi"("cmd"=enum16{"Start", "Finish"}."Finish", "error in"=w458) -> ("error out"=w455:errorcluster)  [unwired: 7 in, 2 out]
                            }
                          }
                          n183 = call "fgv_stop_local.vi"("cmd"=init-r-stop."read", "error in (no error)"=w448) -> ("error out"=w446:errorcluster, "stop"=w447:bool)  [unwired: 8 in]
                        }
                      }
                    }
                    frame #1 {
                      n184 = Increment(x=w482) -> (x+1=w484:i32)
                      n185 = global write "Global 1.vi" "작동회수"(w482) -> ()
                      n186 = call "fgv_rc-config.vi"("cmd"=rw."read") -> ("Testconfig out"=w489:T4)  [unwired: 9 in, 1 out]
                      n187 = Get Date/Time In Seconds() -> (seconds since 1Jan1904=w480:timestamp)
                      n188 = To Double Precision Float(number=w473) -> (double precision float=w471:dbl)
                      n189 = call "Timer - 1.vi"("cmd"=cmd_timer."run") -> ("error out"=w474:errorcluster)  [unwired: 8 in, 2 out]
                      n190 = Unbundle By Name(w489) -> ("ON/OFF 회 수[N]"=w485:dbl)
                      n191 = To Double Precision Float(number=w478) -> (double precision float=w479:dbl)
                      n192 = To Double Precision Float(number=w480) -> (double precision float=w472:dbl)
                      n193 = Subtract(x=w472, y=w479) -> (x-y=w477:dbl)
                      n194 = Subtract(x=w472, y=w471) -> (x-y=w470:dbl)
                      n195 = call "Timer - 1.vi"("error in (no error)"=w474, "cmd"=cmd_timer."update") -> ()  [unwired: 7 in, 3 out]
                      n196 = global write "Global 1.vi" "Elapsed Time 작동"(w477) -> ()
                      n197 = global write "Global 1.vi" "ETime 작동대기"(w470) -> ()
                      n198 = To Long Integer(number=w485) -> (32bit integer=w483:i32)
                      n199 = Greater Or Equal?(x=w484, y=w483) -> (x >= y?=w488:bool)
                      n200 = Compound Arithmetic op=OR(w481, w488) -> (w487:bool)
                    }
                  }
                }
              }
              frame #2 {
              }
            }
          }
          frame "Run 2" {
            n201 = stacked-sequence {
              tunnel: w501 -> [_ w508 _]
              tunnel: [_ w507 _] -> w500
              tunnel: w499 -> [_ w506 _]
              tunnel: [_ w505 _] -> w492
              tunnel: w498 -> [_ w504 _]
              tunnel: w497 -> [_ w503 _]
              tunnel: [_ _ w573] -> w496
              tunnel: [_ _ cmd_runStop."Exit" ("Enum")] -> w495
              tunnel: [_ _ w572] -> w494
              tunnel: w493 -> [_ _ w572]
              frame #0 {
                n202 = call "UI_result.vi"("result"=result."작동") -> ()  [unwired: 10 in, 1 out]
              }
              frame #1 {
                n203 = while {
                  tunnel: w508 -> [w519]
                  tunnel: [w517] -> w505
                  tunnel: w504 -> [w516]
                  shift-right: [w518] -> w507
                  shift-left: w506 -> [w510]
                  shift-right: [w513] -> _
                  shift-left: w503 -> [w515]
                  i -> [w512]
                  stop <- w514 stop-if-true
                  n204 = call "Timer - 1.vi"("error in (no error)"=w510, "cmd"=cmd_timer."init") -> ("error out"=w509:errorcluster)  [unwired: 7 in, 2 out]
                  n205 = stacked-sequence {
                    seq-local: [w520 _] -> [_ w565]
                    tunnel: w519 -> [w524 _]
                    tunnel: [w523 _] -> w518
                    tunnel: w509 -> [w522 _]
                    tunnel: [w520 _] -> w517
                    tunnel: w516 -> [w521 _]
                    tunnel: w515 -> [_ w562]
                    tunnel: [_ w563] -> w514
                    tunnel: [_ w562] -> w513
                    tunnel: w512 -> [_ w558]
                    frame #0 {
                      n206 = for {
                        tunnel: [w528] -> w520
                        tunnel: w521 -> [w530] mode=indexing
                        tunnel: w522 -> [w526]
                        tunnel: [w527] -> w523
                        tunnel: w524 -> [w525]
                        i -> [w529]
                        stop <- w528 stop-if-true
                        # "Group start-Finish"
                        n207 = for {
                          N: w525 -> [_]
                          tunnel: w529 -> [w537]
                          tunnel: w526 -> [w536]
                          tunnel: [w531] -> w527
                          tunnel: w530 -> [w538]
                          tunnel: [w532] -> w528
                          i -> [w535]
                          stop <- w532 stop-if-true
                          n208 = case shown="True" w538 {
                            tunnel: w537 -> [_ w547]
                            tunnel: [w539 w540] -> w533
                            tunnel: w536 -> [w539 w542]
                            tunnel: w535 -> [_ w541]
                            frame False {
                            }
                            frame True {
                              # "Ch start-Finish"
                              n209 = call "sub_ch-start-finish.vi"("cmd"=enum16{"Start", "Finish"}."Start", "error in"=w542, "repeat"=w541, "Ch"=w547) -> ("error out"=w548:errorcluster, "HWseq-array"=w545:T9[])  [unwired: 5 in, 1 out]
                              n210 = for {
                                tunnel: w545 -> [w552] mode=indexing
                                tunnel: w548 -> [w549]
                                tunnel: [w550] -> w543
                                stop <- w553 stop-if-true
                                # "single sequence"
                                n211 = call "sub_hw-seq-all.vi"("error"=w549, "HWseq"=w552) -> ("error out"=w551:errorcluster)  [unwired: 9 in]
                                n212 = call "fgv_stop_local.vi"("cmd"=init-r-stop."read", "error in (no error)"=w551) -> ("error out"=w550:errorcluster, "stop"=w553:bool)  [unwired: 8 in]
                              }
                              n213 = call "sub_ch-start-finish.vi"("cmd"=enum16{"Start", "Finish"}."Finish", "error in"=w543) -> ("error out"=w540:errorcluster)  [unwired: 7 in, 2 out]
                            }
                          }
                          n214 = call "fgv_stop_local.vi"("cmd"=init-r-stop."read", "error in (no error)"=w533) -> ("error out"=w531:errorcluster, "stop"=w532:bool)  [unwired: 8 in]
                        }
                      }
                    }
                    frame #1 {
                      n215 = global write "Global 1.vi" "작동회수"(w558) -> ()
                      n216 = Get Date/Time In Seconds() -> (seconds since 1Jan1904=w571:timestamp)
                      n217 = call "fgv_rc-config.vi"("cmd"=rw."read") -> ("Testconfig out"=w568:T4)  [unwired: 9 in, 1 out]
                      n218 = To Double Precision Float(number=w562) -> (double precision float=w569:dbl)
                      n219 = To Double Precision Float(number=w571) -> (double precision float=w570:dbl)
                      n220 = Unbundle By Name(w568) -> ("3. 작동시간[분]"=w561:dbl)
                      n221 = Subtract(x=w570, y=w569) -> (x-y=w566:dbl)
                      n222 = Multiply(x=w561, y=60.0) -> (x*y=w559:dbl)
                      n223 = call "Timer - 1.vi"("cmd"=cmd_timer."run") -> ("error out"=w555:errorcluster)  [unwired: 8 in, 2 out]
                      n224 = call "Timer - 1.vi"("error in (no error)"=w555, "cmd"=cmd_timer."update") -> ()  [unwired: 7 in, 3 out]
                      n225 = Greater Or Equal?(x=w566, y=w559) -> (x >= y?=w564:bool)
                      n226 = Compound Arithmetic op=OR(w565, w564) -> (w563:bool)
                    }
                  }
                }
              }
              frame #2 {
                n227 = Get Date/Time In Seconds() -> (seconds since 1Jan1904=w573:timestamp)
              }
            }
          }
          frame "Stop" {
            n228 = global write "Glob_setting.vi" "result"(result."작동 대기" ("result")) -> ()
            n229 = call "UI_result.vi"("result"=result."작동 대기", "error in (no error)"=w577) -> ()  [unwired: 9 in, 1 out]
            n230 = stacked-sequence {
              tunnel: w583 -> [w586 _]
              tunnel: [_ w627] -> w582
              tunnel: [w585 _] -> w576
              tunnel: [_ w613] -> w581
              tunnel: w580 -> [w584 w616]
              tunnel: [_ w616] -> w579
              frame #0 {
                n231 = while {
                  tunnel: [w596] -> w585
                  shift-right: [w597] -> _
                  shift-left: w586 -> [w597]
                  tunnel: w584 -> [w590]
                  i -> [w592]
                  stop <- w598 stop-if-true
                  n232 = Get Date/Time In Seconds() -> (seconds since 1Jan1904=w606:timestamp)
                  n233 = To Double Precision Float(number=w597) -> (double precision float=w605:dbl)
                  n234 = To Double Precision Float(number=w590) -> (double precision float=w588:dbl)
                  n235 = To Double Precision Float(number=w606) -> (double precision float=w589:dbl)
                  n236 = Quotient & Remainder(x=w592, y=100) -> (x-y*floor(x/y)=w594:i32)  [unwired: 1 out]
                  n237 = Subtract(x=w589, y=w605) -> (x-y=w591:dbl)
                  n238 = Subtract(x=w589, y=w588) -> (x-y=w587:dbl)
                  n239 = Equal To 0?(x=w594) -> (x = 0?=w593:bool)
                  n240 = call "fgv_rc-config.vi"("cmd"=rw."read") -> ("Testconfig out"=w604:T4)  [unwired: 9 in, 1 out]
                  n241 = case shown="True" w593 {
                    tunnel: w591 -> [_ w610]
                    tunnel: w587 -> [_ w609]
                    frame False {
                    }
                    frame True {
                      n242 = call "Timer.vi"("cmd"=cmd_timer."run") -> ()  [unwired: 8 in, 3 out]
                      n243 = global write "Global 1.vi" "Elapsed Time 작동"(w610) -> ()
                      n244 = global write "Global 1.vi" "ETime 작동대기"(w609) -> ()
                    }
                  }
                  n245 = Unbundle By Name(w604) -> ("1. 작동시간[분]"=w602:dbl)
                  n246 = Multiply(x=w602, y=60.0) -> (x*y=w600:dbl)
                  n247 = Greater Or Equal?(x=w591, y=w600) -> (x >= y?=w599:bool)
                  n248 = call "fgv_stop_local.vi"("cmd"=init-r-stop."read") -> ("stop"=w596:bool)  [unwired: 9 in, 1 out]
                  n249 = Compound Arithmetic op=OR(w596, w599) -> (w598:bool)
                  n250 = Wait (ms)(milliseconds to wait=u32 1) -> ()  [unwired: 1 out]
                }
              }
              frame #1 {
                n251 = call "fgv_rc-config.vi"("cmd"=rw."read") -> ("Testconfig out"=w626:T4)  [unwired: 9 in, 1 out]
                n252 = Unbundle By Name(w626) -> ("시험시간[분]"=w622:dbl)
                n253 = Get Date/Time In Seconds() -> (seconds since 1Jan1904=w620:timestamp)
                n254 = To Double Precision Float(number=w616) -> (double precision float=w618:dbl)
                n255 = To Double Precision Float(number=w622) -> (double precision float=w621:dbl)
                n256 = To Double Precision Float(number=w620) -> (double precision float=w619:dbl)
                n257 = Multiply(x=w621, y=60.0) -> (x*y=w623:dbl)
                n258 = Subtract(x=w619, y=w618) -> (x-y=w617:dbl)
                n259 = Greater Or Equal?(x=w617, y=w623) -> (x >= y?=w615:bool)
                n260 = Select(t=cmd_runStop."Exit" ("Enum"), s=w615, f=cmd_runStop."Run 1" ("Enum")) -> (s? t:f=w613:T2)
                n261 = Get Date/Time In Seconds() -> (seconds since 1Jan1904=w627:timestamp)
              }
            }
          }
          frame "Exit" {
            w628 = timestamp(0 s since 1904-01-01) ("seconds since 1Jan1904")
          }
        }
      }
    }
    frame "6.3.9 빙결 시험" {
      n262 = while {
        tunnel: w637 -> [w650]
        tunnel: w633 -> [w646]
        shift-right: [w649] -> w636
        shift-left: w635 -> [w648]
        shift-right: [w644] -> _
        shift-left: _ -> [w643]
        shift-right: [w642] -> _
        shift-left: w632 -> [w645]
        shift-right: [w647] -> w634
        shift-left: _ -> [w641]
        shift-right: [w639] -> _
        shift-left: _ -> [w638]
        stop <- w640 stop-if-true
        n263 = case shown="\"Run 1\"" w645 {
          tunnel: w650 -> [_ w670 w759 _ _]
          tunnel: [w660 w669 w758 _ _] -> w649
          tunnel: w648 -> [w660 w668 w757 w830 _]
          tunnel: [FALSE ("stop") w661 w750 w829 w886] -> w647
          tunnel: w646 -> [_ w667 w756 _ _]
          tunnel: [w657 w665 w754 w835 w884] -> w644
          tunnel: w643 -> [_ w666 w755 w836 _]
          tunnel: [cmd_runStop."Run 1" ("Enum") w664 w753 w834 cmd_runStop."Init" ("Enum")] -> w642
          tunnel: w641 -> [_ _ _ _ w886]
          tunnel: [_ w661 w750 w829 TRUE] -> w640
          tunnel: [w657 w662 w752 w832 w884] -> w639
          tunnel: w638 -> [_ w663 w751 w833 _]
          frame "Init", Default {
            w651 = 0.0 ("Elapsed Time")
            n264 = global write "Global 1.vi" "Elapsed Time 작동"(w651) -> ()
            n265 = global write "Global 1.vi" "작동회수"(0 ("작동회수")) -> ()
            n266 = global write "Global 1.vi" "스위칭 시간"(w651) -> ()
            n267 = global write "Global 1.vi" "Elapsed Time 미작동"(w651) -> ()
            n268 = global write "Global 1.vi" "ETime 작동대기"(w651) -> ()
            n269 = global read "Global 1.vi" "작동시간(초)"() -> (w655:refnum<vi>)
            n270 = global write "Glob_setting.vi" "result"(result."Init" ("result")) -> ()
            n271 = property class="DigNum (strict)"(reference=w655, "Caption.Text"="작동경과 시간(초)" ("Label.Text")) -> ()  [unwired: 1 in, 2 out]
            n272 = call "Timer - 1.vi"("cmd"=cmd_timer."init_update") -> ()  [unwired: 8 in, 3 out]
            n273 = Get Date/Time In Seconds() -> (seconds since 1Jan1904=w657:timestamp)
          }
          frame "Run 1" {
            n274 = stacked-sequence {
              tunnel: w670 -> [_ w680 _]
              tunnel: [_ w679 _] -> w669
              tunnel: w668 -> [_ w678 _]
              tunnel: [_ w677 _] -> w661
              tunnel: w667 -> [_ w676 _]
              tunnel: w666 -> [_ w675 _]
              tunnel: [_ w674 _] -> w665
              tunnel: [_ _ cmd_runStop."Stop" ("Enum")] -> w664
              tunnel: w663 -> [_ w673 w748]
              tunnel: [_ _ w748] -> w662
              frame #0 {
                n275 = global write "Glob_setting.vi" "result"(result."작동" ("result")) -> ()
                n276 = call "UI_result.vi"("result"=result."작동") -> ()  [unwired: 10 in, 1 out]
              }
              frame #1 {
                n277 = while {
                  tunnel: w680 -> [w692]
                  tunnel: [w690] -> w677
                  tunnel: w676 -> [w689]
                  shift-right: [w691] -> w679
                  shift-left: w678 -> [w683]
                  shift-right: [w686] -> w674
                  shift-left: w675 -> [w688]
                  tunnel: w673 -> [w681]
                  i -> [w685]
                  stop <- w687 stop-if-true
                  n278 = call "Timer - 1.vi"("error in (no error)"=w683, "cmd"=cmd_timer."init") -> ("error out"=w682:errorcluster)  [unwired: 7 in, 2 out]
                  n279 = stacked-sequence {
                    seq-local: [w693 _] -> [_ w746]
                    tunnel: w692 -> [w697 _]
                    tunnel: [w696 _] -> w691
                    tunnel: w682 -> [w695 _]
                    tunnel: [w693 _] -> w690
                    tunnel: w689 -> [w694 _]
                    tunnel: w688 -> [_ w737]
                    tunnel: [_ TRUE] -> w687
                    tunnel: [_ w737] -> w686
                    tunnel: w685 -> [_ w739]
                    tunnel: w681 -> [_ w731]
                    frame #0 {
                      n280 = for {
                        tunnel: [w701] -> w693
                        tunnel: w694 -> [w703] mode=indexing
                        tunnel: w695 -> [w699]
                        tunnel: [w700] -> w696
                        tunnel: w697 -> [w698]
                        i -> [w702]
                        stop <- w701 stop-if-true
                        # "Group start-Finish"
                        n281 = for {
                          N: w698 -> [_]
                          tunnel: w702 -> [w710]
                          tunnel: w699 -> [w709]
                          tunnel: [w704] -> w700
                          tunnel: w703 -> [w711]
                          tunnel: [w705] -> w701
                          i -> [w708]
                          stop <- w705 stop-if-true
                          n282 = case shown="True" w711 {
                            tunnel: w710 -> [_ w720]
                            tunnel: [w712 w713] -> w706
                            tunnel: w709 -> [w712 w715]
                            tunnel: w708 -> [_ w714]
                            frame False {
                            }
                            frame True {
                              # "Ch start-Finish"
                              n283 = call "sub_ch-start-finish.vi"("cmd"=enum16{"Start", "Finish"}."Start", "error in"=w715, "repeat"=w714, "Ch"=w720) -> ("error out"=w721:errorcluster, "HWseq-array"=w718:T9[])  [unwired: 5 in, 1 out]
                              n284 = for {
                                tunnel: w718 -> [w725] mode=indexing
                                tunnel: w721 -> [w722]
                                tunnel: [w723] -> w716
                                stop <- w726 stop-if-true
                                # "single sequence"
                                n285 = call "sub_hw-seq-all.vi"("error"=w722, "HWseq"=w725) -> ("error out"=w724:errorcluster)  [unwired: 9 in]
                                n286 = call "fgv_stop_local.vi"("cmd"=init-r-stop."read", "error in (no error)"=w724) -> ("error out"=w723:errorcluster, "stop"=w726:bool)  [unwired: 8 in]
                              }
                              n287 = call "sub_ch-start-finish.vi"("cmd"=enum16{"Start", "Finish"}."Finish", "error in"=w716) -> ("error out"=w713:errorcluster)  [unwired: 7 in, 2 out]
                            }
                          }
                          n288 = call "fgv_stop_local.vi"("cmd"=init-r-stop."read", "error in (no error)"=w706) -> ("error out"=w704:errorcluster, "stop"=w705:bool)  [unwired: 8 in]
                        }
                      }
                    }
                    frame #1 {
                      n289 = Increment(x=w739) -> (x+1=w742:i32)
                      n290 = global write "Global 1.vi" "작동회수"(w739) -> ()
                      n291 = call "fgv_rc-config.vi"("cmd"=rw."read") -> ("Testconfig out"=w747:T4)  [unwired: 9 in, 1 out]
                      n292 = call "Timer - 1.vi"("cmd"=cmd_timer."run") -> ("error out"=w733:errorcluster)  [unwired: 8 in, 2 out]
                      n293 = Unbundle By Name(w747) -> ("ON/OFF 회 수[N]"=w743:dbl)
                      n294 = Get Date/Time In Seconds() -> (seconds since 1Jan1904=w738:timestamp)
                      n295 = To Double Precision Float(number=w731) -> (double precision float=w729:dbl)
                      n296 = To Double Precision Float(number=w737) -> (double precision float=w732:dbl)
                      n297 = call "Timer - 1.vi"("error in (no error)"=w733, "cmd"=cmd_timer."update") -> ()  [unwired: 7 in, 3 out]
                      n298 = To Double Precision Float(number=w738) -> (double precision float=w730:dbl)
                      n299 = Subtract(x=w730, y=w732) -> (x-y=w736:dbl)
                      n300 = Subtract(x=w730, y=w729) -> (x-y=w728:dbl)
                      n301 = To Long Integer(number=w743) -> (32bit integer=w741:i32)
                      n302 = global write "Global 1.vi" "Elapsed Time 작동"(w736) -> ()
                      n303 = global write "Global 1.vi" "ETime 작동대기"(w728) -> ()
                      n304 = Greater Or Equal?(x=w742, y=w741) -> (x >= y?=w745:bool)
                      n305 = Compound Arithmetic op=OR(w746, w745) -> ()  [unwired: 1 out]
                    }
                  }
                }
              }
              frame #2 {
              }
            }
          }
          frame "Run 2" {
            n306 = stacked-sequence {
              tunnel: w759 -> [_ w766 _]
              tunnel: [_ w765 _] -> w758
              tunnel: w757 -> [_ w764 _]
              tunnel: [_ w763 _] -> w750
              tunnel: w756 -> [_ w762 _]
              tunnel: w755 -> [_ w761 _]
              tunnel: [_ _ w826] -> w754
              tunnel: [_ _ cmd_runStop."Exit" ("Enum")] -> w753
              tunnel: [_ _ w825] -> w752
              tunnel: w751 -> [_ _ w825]
              frame #0 {
                n307 = call "UI_result.vi"("result"=result."작동") -> ()  [unwired: 10 in, 1 out]
              }
              frame #1 {
                n308 = while {
                  tunnel: w766 -> [w775]
                  tunnel: [w772] -> w763
                  tunnel: w762 -> [w771]
                  shift-right: [w774] -> w765
                  shift-left: w764 -> [w773]
                  shift-right: [w768] -> _
                  shift-left: w761 -> [w770]
                  i -> [w767]
                  stop <- w769 stop-if-true
                  n309 = stacked-sequence {
                    seq-local: [w776 _] -> [_ w818]
                    tunnel: w775 -> [w780 _]
                    tunnel: [w779 _] -> w774
                    tunnel: w773 -> [w778 _]
                    tunnel: [w776 _] -> w772
                    tunnel: w771 -> [w777 _]
                    tunnel: w770 -> [_ w815]
                    tunnel: [_ w816] -> w769
                    tunnel: [_ w815] -> w768
                    tunnel: w767 -> [_ w811]
                    frame #0 {
                      n310 = for {
                        tunnel: [w784] -> w776
                        tunnel: w777 -> [w786] mode=indexing
                        tunnel: w778 -> [w782]
                        tunnel: [w783] -> w779
                        tunnel: w780 -> [w781]
                        i -> [w785]
                        stop <- w784 stop-if-true
                        # "Group start-Finish"
                        n311 = for {
                          N: w781 -> [_]
                          tunnel: w785 -> [w793]
                          tunnel: w782 -> [w792]
                          tunnel: [w787] -> w783
                          tunnel: w786 -> [w794]
                          tunnel: [w788] -> w784
                          i -> [w791]
                          stop <- w788 stop-if-true
                          n312 = case shown="True" w794 {
                            tunnel: w793 -> [_ w803]
                            tunnel: [w795 w796] -> w789
                            tunnel: w792 -> [w795 w798]
                            tunnel: w791 -> [_ w797]
                            frame False {
                            }
                            frame True {
                              # "Ch start-Finish"
                              n313 = call "sub_ch-start-finish.vi"("cmd"=enum16{"Start", "Finish"}."Start", "error in"=w798, "repeat"=w797, "Ch"=w803) -> ("error out"=w804:errorcluster, "HWseq-array"=w801:T9[])  [unwired: 5 in, 1 out]
                              n314 = for {
                                tunnel: w801 -> [w808] mode=indexing
                                tunnel: w804 -> [w805]
                                tunnel: [w806] -> w799
                                stop <- w809 stop-if-true
                                # "single sequence"
                                n315 = call "sub_hw-seq-all.vi"("error"=w805, "HWseq"=w808) -> ("error out"=w807:errorcluster)  [unwired: 9 in]
                                n316 = call "fgv_stop_local.vi"("cmd"=init-r-stop."read", "error in (no error)"=w807) -> ("error out"=w806:errorcluster, "stop"=w809:bool)  [unwired: 8 in]
                              }
                              n317 = call "sub_ch-start-finish.vi"("cmd"=enum16{"Start", "Finish"}."Finish", "error in"=w799) -> ("error out"=w796:errorcluster)  [unwired: 7 in, 2 out]
                            }
                          }
                          n318 = call "fgv_stop_local.vi"("cmd"=init-r-stop."read", "error in (no error)"=w789) -> ("error out"=w787:errorcluster, "stop"=w788:bool)  [unwired: 8 in]
                        }
                      }
                    }
                    frame #1 {
                      n319 = global write "Global 1.vi" "작동회수"(w811) -> ()
                      n320 = Get Date/Time In Seconds() -> (seconds since 1Jan1904=w824:timestamp)
                      n321 = call "fgv_rc-config.vi"("cmd"=rw."read") -> ("Testconfig out"=w821:T4)  [unwired: 9 in, 1 out]
                      n322 = To Double Precision Float(number=w815) -> (double precision float=w822:dbl)
                      n323 = To Double Precision Float(number=w824) -> (double precision float=w823:dbl)
                      n324 = Unbundle By Name(w821) -> ("3. 작동시간[분]"=w814:dbl)
                      n325 = Subtract(x=w823, y=w822) -> (x-y=w819:dbl)
                      n326 = Multiply(x=w814, y=60.0) -> (x*y=w812:dbl)
                      n327 = Greater Or Equal?(x=w819, y=w812) -> (x >= y?=w817:bool)
                      n328 = Compound Arithmetic op=OR(w818, w817) -> (w816:bool)
                    }
                  }
                }
              }
              frame #2 {
                n329 = Get Date/Time In Seconds() -> (seconds since 1Jan1904=w826:timestamp)
              }
            }
          }
          frame "Stop" {
            n330 = global write "Glob_setting.vi" "result"(result."작동 대기" ("result")) -> ()
            n331 = call "UI_result.vi"("result"=result."작동 대기", "error in (no error)"=w830) -> ()  [unwired: 9 in, 1 out]
            n332 = stacked-sequence {
              tunnel: w836 -> [w839 _]
              tunnel: [_ w883] -> w835
              tunnel: [w838 _] -> w829
              tunnel: [_ w870] -> w834
              tunnel: w833 -> [w837 w872]
              tunnel: [_ w872] -> w832
              frame #0 {
                n333 = while {
                  tunnel: [w850] -> w838
                  shift-right: [w843] -> _
                  shift-left: w839 -> [w843]
                  tunnel: w837 -> [w840]
                  i -> [w849]
                  stop <- w851 stop-if-true
                  n334 = call "fgv_rc-config.vi"("cmd"=rw."read") -> ("Testconfig out"=w857:T4)  [unwired: 9 in, 1 out]
                  n335 = Get Date/Time In Seconds() -> (seconds since 1Jan1904=w859:timestamp)
                  n336 = To Double Precision Float(number=w843) -> (double precision float=w858:dbl)
                  n337 = To Double Precision Float(number=w840) -> (double precision float=w844:dbl)
                  n338 = To Double Precision Float(number=w859) -> (double precision float=w842:dbl)
                  n339 = Unbundle By Name(w857) -> ("1. 작동시간[분]"=w855:dbl)
                  n340 = Subtract(x=w842, y=w844) -> (x-y=w841:dbl)
                  n341 = Subtract(x=w842, y=w858) -> (x-y=w845:dbl)
                  n342 = Quotient & Remainder(x=w849, y=100) -> (x-y*floor(x/y)=w847:i32)  [unwired: 1 out]
                  n343 = Equal To 0?(x=w847) -> (x = 0?=w846:bool)
                  n344 = case shown="True" w846 {
                    tunnel: w845 -> [_ w863]
                    tunnel: w841 -> [_ w862]
                    frame False {
                    }
                    frame True {
                      n345 = call "Timer.vi"("cmd"=cmd_timer."run") -> ()  [unwired: 8 in, 3 out]
                      n346 = global write "Global 1.vi" "Elapsed Time 작동"(w863) -> ()
                      n347 = global write "Global 1.vi" "ETime 작동대기"(w862) -> ()
                    }
                  }
                  n348 = Multiply(x=w855, y=60.0) -> (x*y=w853:dbl)
                  n349 = Greater Or Equal?(x=w845, y=w853) -> (x >= y?=w852:bool)
                  n350 = call "fgv_stop_local.vi"("cmd"=init-r-stop."read") -> ("stop"=w850:bool)  [unwired: 9 in, 1 out]
                  n351 = Compound Arithmetic op=OR(w850, w852) -> (w851:bool)
                  n352 = Wait (ms)(milliseconds to wait=u32 1) -> ()  [unwired: 1 out]
                }
              }
              frame #1 {
                n353 = call "fgv_rc-config.vi"("cmd"=rw."read") -> ("Testconfig out"=w882:T4)  [unwired: 9 in, 1 out]
                n354 = Unbundle By Name(w882) -> ("시험시간[분]"=w878:dbl)
                n355 = Get Date/Time In Seconds() -> (seconds since 1Jan1904=w876:timestamp)
                n356 = To Double Precision Float(number=w872) -> (double precision float=w874:dbl)
                n357 = To Double Precision Float(number=w878) -> (double precision float=w877:dbl)
                n358 = To Double Precision Float(number=w876) -> (double precision float=w875:dbl)
                n359 = Multiply(x=w877, y=60.0) -> (x*y=w879:dbl)
                n360 = Subtract(x=w875, y=w874) -> (x-y=w873:dbl)
                n361 = call "fgv_stop_local.vi"("cmd"=init-r-stop."read") -> ("stop"=w867:bool)  [unwired: 9 in, 1 out]
                n362 = Greater Or Equal?(x=w873, y=w879) -> (x >= y?=w866:bool)
                n363 = Compound Arithmetic op=OR(w867, w866) -> (w865:bool)
                n364 = Select(t=cmd_runStop."Exit" ("Enum"), s=w865, f=cmd_runStop."Run 1" ("Enum")) -> (s? t:f=w870:T2)
                n365 = Get Date/Time In Seconds() -> (seconds since 1Jan1904=w883:timestamp)
              }
            }
          }
          frame "Exit" {
            w884 = timestamp(0 s since 1904-01-01) ("seconds since 1Jan1904")
          }
        }
      }
    }
  }
  "error out" <- w10
  "stop" <- w8
